vi "Voltage to Pressure.vi"(11 "AI":dbl) -> (3 "Pressure [mmHg]":dbl)   [LabVIEW 2013]
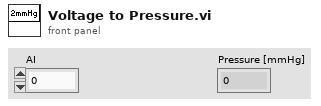
[diagram p1: front panel]
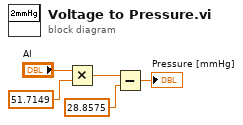
[diagram p0: block diagram]
diagram:
  n1 = Multiply(x="AI", y=51.7149) -> (x*y=w3:dbl)
  n2 = Subtract(x=w3, y=28.8575) -> (x-y=→"Pressure [mmHg]":dbl)
